vi "Create triangles mesh.vi"(2 "Colour":T2={"Red"=1.0, "Green"=1.0, "Blue"=1.0, "Alpha"=1.0}, 3 "Render mode":T3(ring)=enum."Polygons", 4 "Triangles array":T1[](array[typedef])) -> (0 "Error out":errorcluster, 1 "Triangle mesh out":refnum<vi>)   [LabVIEW 2016]
uses:
  <vilib>/Utility/miscctls.llb/LVRGBAColorTypeDef.ctl
  Typedefs/Triangle.ctl
  <vilib>/Utility/miscctls.llb/LV3DPointTypeDef.ctl
  <vilib>/picture/3D Picture Control/Object/Create Object (drawable).vi
  <vilib>/picture/3D Picture Control/NI_3D Picture Control.lvlib
panel:
  # "PN 19/01/2015"
  # "Vertices"
  # "Edges"
  # "Unit normal"
  # "Edge unit normals"
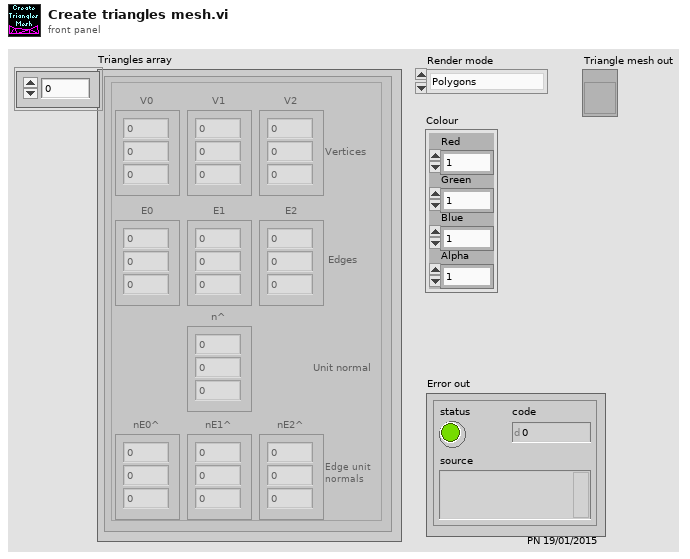
[diagram p1: front panel]
types:
  T1 = typedef "Triangle.ctl" = cluster{"V0":sgl[], "V1":sgl[], "V2":sgl[], "E0":sgl[], "E1":sgl[], "E2":sgl[], "n^":sgl[], "nE0^":sgl[], "nE1^":sgl[], "nE2^":sgl[]}
  T2 = typedef "LVRGBAColorTypeDef.ctl" = cluster{"Red":sgl, "Green":sgl, "Blue":sgl, "Alpha":sgl}
  T3 = enum16{"Inherit Value", "Points", "Wireframe", "Polygons"}
  T4 = enum16{"Inherit Material", "Use entire Material", "Ignore Ambient", "Ignore Diffuse", "Ignore Specular", "Ignore Emission", "Ignore Ambient and Diffuse"}
  T5 = enum16{"Overall", "Per Primitive", "Per Vertex", "Binding Off"}
  T6 = enum16{"Points", "Lines", "Line Strip", "Line Loop", "Triangles", "Triangle Strip", "Triangle Fan", "Quads", "Quad Strip", "Polygon"}
  T7 = enum16{"Inherit Value", "No Culling", "Cull Back Face", "Cull Front Face", "Cull Both Faces"}
  T8 = enum16{"Inherit Value", "Counterclockwise", "Clockwise"}
  T9 = typedef "LV3DPointTypeDef.ctl" = cluster{"X":sgl, "Y":sgl, "Z":sgl}
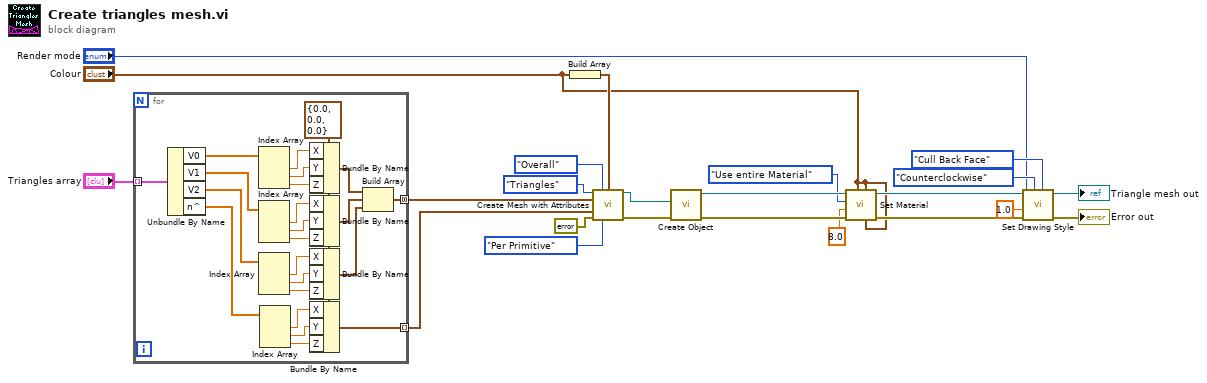
[diagram p0: block diagram]
diagram:
  n1 = for {
    tunnel: "Triangles array" -> [w46] mode=indexing
    tunnel: [w30] -> w15 mode=concatenating
    tunnel: [w25] -> w14 mode=indexing
    w24 = T9 {"X"=0.0, "Y"=0.0, "Z"=0.0} ("3D Point")
    n2 = Unbundle By Name(w46) -> ("V0"=w45:sgl[], "V1"=w44:sgl[], "V2"=w43:sgl[], "n^"=w27:sgl[])
    n3 = Index Array(array=w45) -> (element #1=w42:sgl, element #2=w40:sgl, element #3=w41:sgl)  [unwired: 3 in]
    n4 = Index Array(array=w44) -> (element #1=w39:sgl, element #2=w38:sgl, element #3=w37:sgl)  [unwired: 3 in]
    n5 = Index Array(array=w43) -> (element #1=w36:sgl, element #2=w35:sgl, element #3=w34:sgl)  [unwired: 3 in]
    n6 = Index Array(array=w27) -> (element #1=w26:sgl, element #2=w28:sgl, element #3=w29:sgl)  [unwired: 3 in]
    n7 = Bundle By Name(cluster=w24, "X"=w42, "Y"=w40, "Z"=w41) -> (w33:T9)
    n8 = Bundle By Name(cluster=w24, "X"=w39, "Y"=w38, "Z"=w37) -> (w32:T9)
    n9 = Bundle By Name(cluster=w24, "X"=w36, "Y"=w35, "Z"=w34) -> (w31:T9)
    n10 = Bundle By Name(cluster=w24, "X"=w26, "Y"=w28, "Z"=w29) -> (w25:T9)
    n11 = Build Array(w33, w32, w31) -> (w30:T9[])
  }
  n12 = Build Array("Colour") -> (w3:T2[])
  n13 = call <vilib>:"Create Mesh with Attributes.vi"("Draw Mode"=T6."Triangles", "Color Binding Mode"=T5."Overall", "Color Array"=w3, "Vertex Array"=w15, "Normal Array"=w14, "error in (no error)"=errorcluster {"status"=FALSE, "code"=0, "source"=""}, "Normal Binding Mode"=T5."Per Primitive") -> ("New Mesh Refnum"=w17:refnum<vi>, "error out"=w18:errorcluster)  [unwired: 7 in]
  n14 = call-poly <vilib>:"Create Object.vi"("error in (no error)"=w18, "Geometry"=w17) -> ("error out"=w6:errorcluster, "Scene:New Object"=w8:refnum<vi>)  [unwired: 8 in]
  n15 = call <vilib>:"Set Material.vi"("Diffuse"="Colour", "Specular"="Colour", "Ambient"="Colour", "error in (no error)"=w6, "Shininess"=sgl 8.0, "Color Mode"=T4."Use entire Material", "Scene Object In"=w8) -> ("error out"=w5:errorcluster, "Scene Object Out"=w7:refnum<vi>)  [unwired: 3 in]
  n16 = call <vilib>:"Set Drawing Style.vi"("Face Culling Mode"=T7."Cull Back Face", "Frontface Mode"=T8."Counterclockwise", "error in (no error)"=w5, "Size"=1.0, "Mode"="Render mode", "Scene Object In"=w7) -> ("error out"=→"Error out":errorcluster, "Scene Object Out"=→"Triangle mesh out":refnum<vi>)  [unwired: 4 in]
